vi "03TRM800_GetScopeshot2.vi"() -> ()   [LabVIEW 2015]
panel:
  out "String":string
  out "Array":u16[](array[numeric])
  out "element":bool
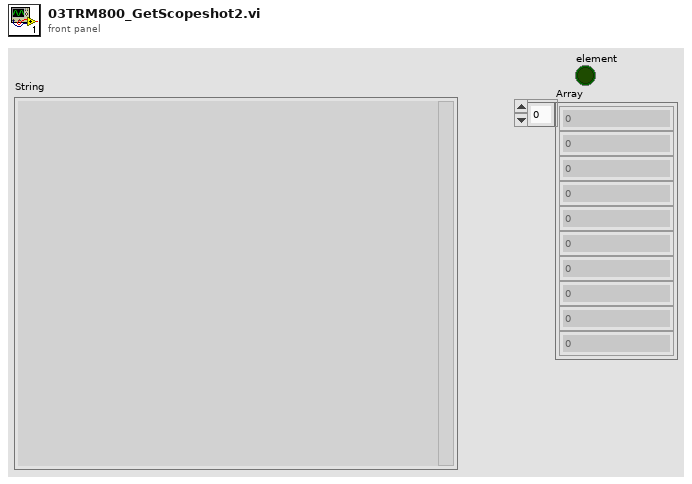
[diagram p1: front panel]
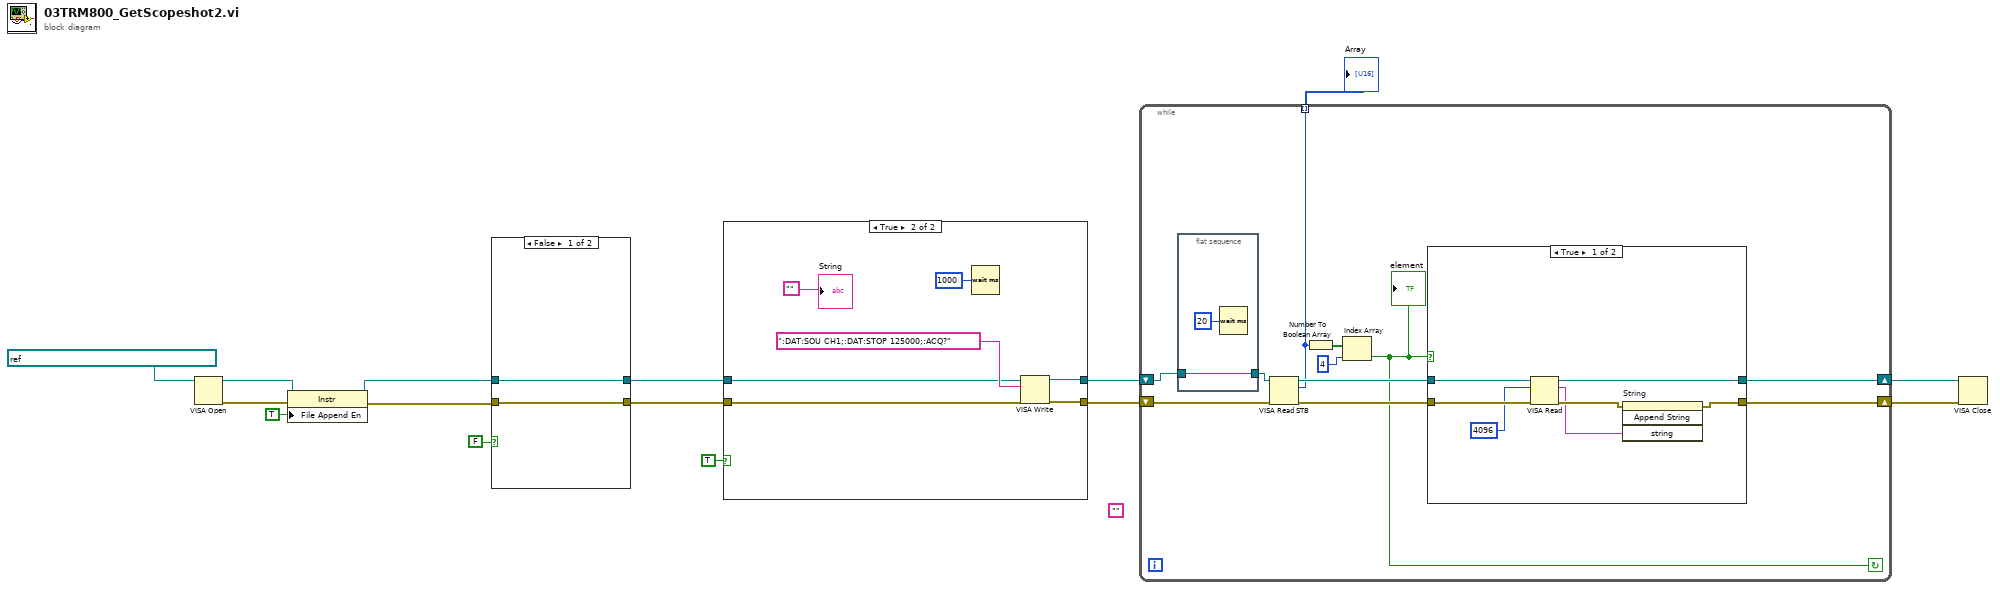
[diagram p0: block diagram]
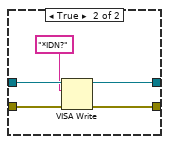
[diagram p4: hidden frame]
diagram:
  (unwired) ""
  n1 = VISA Open(VISA resource name=refnum<visa-resource-name> "USB0::0x0699::0x03A3::C030457::INSTR") -> (VISA resource name=w4:refnum<visa-resource-name>, error out=w5:errorcluster)  [unwired: 4 in]
  n2 = property class="Instr"(reference=w4, error in=w5, "File Append En"=TRUE ("Message Based Settings:File Append Enable")) -> (reference out=w3:refnum<visa-resource-name>, error out=w2:errorcluster)
  n3 = case shown="False" FALSE {
    tunnel: [w17 w20] -> w11
    tunnel: w3 -> [w17 w22]
    tunnel: [w16 w19] -> w10
    tunnel: w2 -> [w16 w21]
    frame False {
    }
    frame True {
      n4 = VISA Write(VISA resource name=w22, write buffer="*IDN?", error in (no error)=w21) -> (VISA resource name out=w20:refnum<visa-resource-name>, error out=w19:errorcluster)  [unwired: 1 out]
    }
  }
  n5 = case shown="True" TRUE {
    tunnel: w11 -> [w24 w26]
    tunnel: w10 -> [w23 w25]
    tunnel: [w24 w30] -> w9
    tunnel: [w23 w31] -> w8
    frame False {
    }
    frame True {
      n6 = Wait (ms)(milliseconds to wait=u32 1000) -> ()  [unwired: 1 out]
      n7 = VISA Write(VISA resource name=w26, write buffer=":DAT:SOU CH1;:DAT:STOP 125000;:ACQ?", error in (no error)=w25) -> (VISA resource name out=w30:refnum<visa-resource-name>, error out=w31:errorcluster)  [unwired: 1 out]
      "String" <- ""
    }
  }
  n8 = while {
    shift-right: [w39] -> w13
    shift-left: w9 -> [w33]
    shift-right: [w38] -> w12
    shift-left: w8 -> [w42]
    tunnel: [w32] -> w6 mode=indexing
    stop <- w35 continue-if-true
    n9 = flat-sequence {
      tunnel: [w44] -> w34
      tunnel: w33 -> [w44]
      frame #0 {
        n10 = Wait (ms)(milliseconds to wait=u32 20) -> ()  [unwired: 1 out]
      }
    }
    n11 = VISA Read STB(8:w42, 11:w34) -> (0:w40:errorcluster, 2:w32:u16, 3:w41:refnum<visa-resource-name>)
    n12 = Number To Boolean Array(number=w32) -> (Boolean array=w37:bool[])
    n13 = Index Array(array=w37, index=4) -> (element=w35:bool)
    "element" <- w35
    n14 = case shown="True" w35 {
      tunnel: w41 -> [w51 w53]
      tunnel: w40 -> [w50 w52]
      tunnel: [w48 w53] -> w39
      tunnel: [w46 w52] -> w38
      frame True {
        n15 = VISA Read(VISA resource name=w51, byte count=u32 4096, error in (no error)=w50) -> (VISA resource name out=w48:refnum<visa-resource-name>, read buffer=w45:string, error out=w47:errorcluster)  [unwired: 1 out]
        n16 = invoke on="String" class="Str" method="Append String"(error in=w47, "string"=w45) -> (error out=w46:errorcluster)  [unwired: 2 in, 3 out]
      }
      frame False {
      }
    }
  }
  "Array" <- w6
  n17 = VISA Close(VISA resource name=w13, error in (no error)=w12) -> ()  [unwired: 1 out]
